vi "FX_Config Extract All.vi"(6 "Send Cmd Timout(ms)":u32=300, 8 "Error":errorcluster, 10 "FX Config":T1={"CAN"={"ID"=0, "Bus"=""}, "Output"={"Inverted"=FALSE, "Neutral"=enum."Override to Coast", "Max"={"FWD"=1.0, "REV"=-1.0}, "Min"={"FWD"=0.0, "REV"=0.0}, "OL Ramp Rate (S)"=0.0, "Dead Band"=0.0, "CL Ramp Rate (S)"=0.0}, "CL"={"Gains"={"P"=1.0, "I"=0.01, "D"=0.0, "F"=0.0}, "Error Allowed"={"High"=0.0, "Low"=0.0}, "I Zone"={"High"=10000.0, "Low"=-1000.0}, "Max Out"={"FWD"=1.0, "REV"=-1.0}, "Max I Accu"={"High"=10.0, "Low"=-10.0}, "CL Ramp Rate (S)"=0.0}, "MM"={"Cruise Velocity"=5000, "Acceleration"=5000}, "TravelLimits"={"Hard"={"FWD Switch Normal"=enum."Normally Open", "FWD On will Zero Encoder "=FALSE, "REV Switch Normal"=enum."Normally Open", "REV On will Zero Encoder "=FALSE}, "Soft"={"FWD"={"Enable"=FALSE, "Counts"=0}, "REV"={"Enable"=FALSE, "Counts"=0}}}, "CurrentLimit"={"Enable"=FALSE, "Current Limit"=0.0, "Threshold Current"=0.0, "Threshold Time"=0.0}} {"TravelLimits"."Soft"."REV"."Counts" format="%#.0f"; "TravelLimits"."Soft"."FWD"."Counts" format="%#.0f"; "Output"."Min"."REV" format="%.2f"; "Output"."Min"."FWD" format="%.2f"; "Output"."Max"."REV" format="%.2f"; "Output"."Max"."FWD" format="%.2f"; "CL"."Max I Accu"."Low" format="%#.8f"; "CL"."Max I Accu"."High" format="%#.8f"; "CL"."Gains"."F" format="%#.8f"; "CL"."Gains"."D" format="%#.8f"; "CL"."Gains"."I" format="%#.8f"; "CL"."Gains"."P" format="%#.8f"; "CL"."Error Allowed"."Low" format="%#.8f"; "CL"."Error Allowed"."High" format="%#.8f"; "CL"."I Zone"."Low" format="%#.8f"; "CL"."I Zone"."High" format="%#.8f"; "CL"."Max Out"."REV" format="%.2f"; "CL"."Max Out"."FWD" format="%.2f"}, 11 "PhoenixMotorControlDevRef":T16={"DeviceStatus"={"status"=FALSE, "code"=0, "source"=""}, "Type"=enum."PWM", "PWM"={"PWM Channel"=enum."Invalid", "DeadBand"={"Name"="", "maxPositivePwm"=0, "minPositivePwm"=0, "centerPwm"=0, "maxNegativePwm"=0, "minNegativePwm"=0, "angularRange"=0}}, "CAN"={"Device Number"=0, "SetOutput VI Ref"=variant, "GetOutput VI Ref"=variant, "Enable VI Ref"=variant, "Disable VI Ref"=variant, "Data"=variant}, "Invert"=FALSE, "DIO PWM"={"PWM \"Enable\" Channel"=enum."Invalid", "DIOChannel"=enum."Invalid", "PWM Rate"=0.0}}) -> (0 "Error Out":errorcluster, 2 "Wrist Config Data Out":T1={"CAN"={"ID"=0, "Bus"=""}, "Output"={"Inverted"=FALSE, "Neutral"=enum."Override to Coast", "Max"={"FWD"=1.0, "REV"=-1.0}, "Min"={"FWD"=0.0, "REV"=0.0}, "OL Ramp Rate (S)"=0.0, "Dead Band"=0.0, "CL Ramp Rate (S)"=0.0}, "CL"={"Gains"={"P"=1.0, "I"=0.01, "D"=0.0, "F"=0.0}, "Error Allowed"={"High"=0.0, "Low"=0.0}, "I Zone"={"High"=10000.0, "Low"=-1000.0}, "Max Out"={"FWD"=1.0, "REV"=-1.0}, "Max I Accu"={"High"=10.0, "Low"=-10.0}, "CL Ramp Rate (S)"=0.0}, "MM"={"Cruise Velocity"=5000, "Acceleration"=5000}, "TravelLimits"={"Hard"={"FWD Switch Normal"=enum."Normally Open", "FWD On will Zero Encoder "=FALSE, "REV Switch Normal"=enum."Normally Open", "REV On will Zero Encoder "=FALSE}, "Soft"={"FWD"={"Enable"=FALSE, "Counts"=0}, "REV"={"Enable"=FALSE, "Counts"=0}}}, "CurrentLimit"={"Enable"=FALSE, "Current Limit"=0.0, "Threshold Current"=0.0, "Threshold Time"=0.0}} {"TravelLimits"."Soft"."REV"."Counts" format="%#.0f"; "TravelLimits"."Soft"."FWD"."Counts" format="%#.0f"; "Output"."Min"."REV" format="%.2f"; "Output"."Min"."FWD" format="%.2f"; "Output"."Max"."REV" format="%.2f"; "Output"."Max"."FWD" format="%.2f"; "CL"."Max I Accu"."Low" format="%#.8f"; "CL"."Max I Accu"."High" format="%#.8f"; "CL"."Gains"."F" format="%#.8f"; "CL"."Gains"."D" format="%#.8f"; "CL"."Gains"."I" format="%#.8f"; "CL"."Gains"."P" format="%#.8f"; "CL"."Error Allowed"."Low" format="%#.8f"; "CL"."Error Allowed"."High" format="%#.8f"; "CL"."I Zone"."Low" format="%#.8f"; "CL"."I Zone"."High" format="%#.8f"; "CL"."Max Out"."REV" format="%.2f"; "CL"."Max Out"."FWD" format="%.2f"}, 3 "Module Azimuth Ref Out":T16)   [LabVIEW 2020]
uses:
  <vilib>/Utility/Data Type/NI_Data Type.lvlib
  <vilib>/Rock Robotics/WPI/ThirdParty/Phoenix-LabVIEW/Motor Controller/Controls/CTRE_Phoenix_MotorControl_LimitSwitchNormal.ctl
  <vilib>/Rock Robotics/WPI/ThirdParty/Phoenix-LabVIEW/Motor Controller/Controls/CTRE_Phoenix_MotorControl_TalonFXInvertType.ctl
  <vilib>/Rock Robotics/WPI/ThirdParty/Phoenix-LabVIEW/Motor Controller/Controls/CTRE_Phoenix_MotorControl_NeutralMode.ctl
  Shared Code/TypeDefs/Cluser_CAN Data.ctl
  Shared Code/TypeDefs/Cluster_FWD  REV Values.ctl
  Shared Code/TypeDefs/Cluster_Config SRX Motor Output.ctl
  Shared Code/TypeDefs/Cluster_PID Gains.ctl
  Shared Code/TypeDefs/Cluster_SRX SLOT PID Config.ctl
  Shared Code/TypeDefs/Cluster_SRX Motion Magic Parameters.ctl
  Shared Code/TypeDefs/Cluser_Hard Limits.ctl
  Shared Code/TypeDefs/Cluser_Enable-Value I32.ctl
  Shared Code/TypeDefs/Cluser_Config_Soft Limits.ctl
  Shared Code/TypeDefs/Cluser_Limit Travel Config.ctl
  Shared Code/TypeDefs/Cluster_Cancoder_Config Data.ctl
  <vilib>/Rock Robotics/SystemInterfaces/DIO/FPGA_DIOPWMChannel.ctl
  <vilib>/Rock Robotics/WPI/PWM/WPI_PWMDeadband.ctl
  <vilib>/Rock Robotics/WPI/MotorControl/WPI_MotorControlType.ctl
  <vilib>/Rock Robotics/SystemInterfaces/DIO/FPGA_DIOChannel.ctl
  <vilib>/Rock Robotics/WPI/MotorControl/WPI_MotorControlDeviceRef.ctl
  Shared Code/TypeDefs/Cluster_High-Low.ctl
  Shared Code/TypeDefs/Cluser_Config_Current Limits.ctl
  Shared Code/TypeDefs/Cluster_FX Config HW Values.ctl
panel:
  # "Tune Output\nto 1023 Max"
  # "Tune Output\nto 1023 Max"
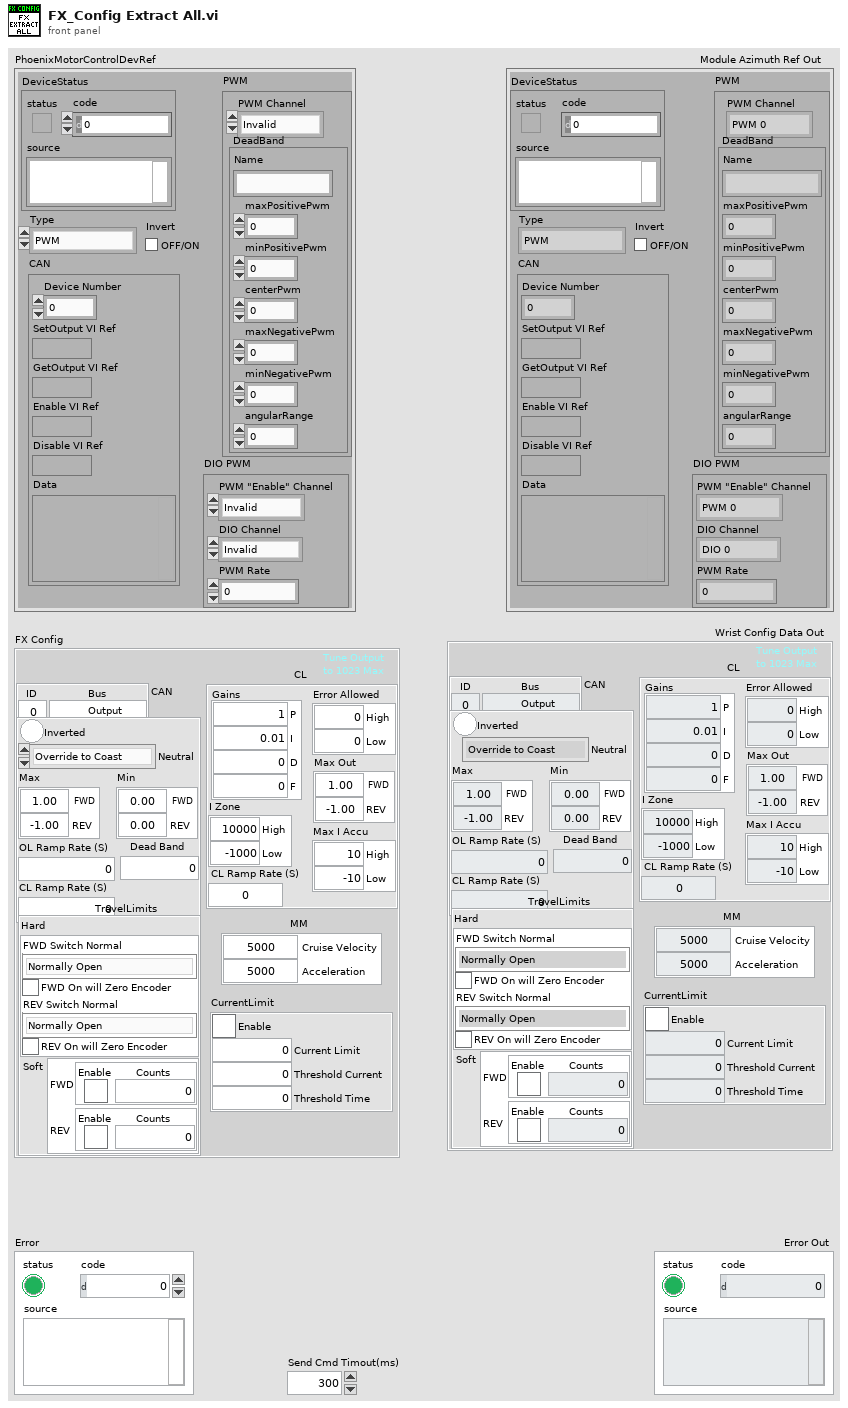
[diagram p1: front panel]
types:
  T1 = typedef "Cluster_FX Config HW Values.ctl" = cluster{"CAN":T2, "Output":T3, "CL":T6, "MM":T9, "TravelLimits":T10, "CurrentLimit":T15}
  T2 = typedef "Cluser_CAN Data.ctl" = cluster{"ID":u8, "Bus":string}
  T3 = typedef "Cluster_Config SRX Motor Output.ctl" = cluster{"Inverted":bool, "Neutral":T4, "Max":T5, "Min":T5, "OL Ramp Rate (S)":dbl, "Dead Band":dbl, "CL Ramp Rate (S)":dbl}
  T4 = typedef "CTRE_Phoenix_MotorControl_NeutralMode.ctl" = enum8{"EEPROMSetting", "Override to Coast", "Override to Brake"}
  T5 = typedef "Cluster_FWD  REV Values.ctl" = cluster{"FWD":dbl, "REV":dbl}
  T6 = typedef "Cluster_PID Config.ctl" = cluster{"Gains":T7, "Error Allowed":T8, "I Zone":T8, "Max Out":T5, "Max I Accu":T8, "CL Ramp Rate (S)":dbl}
  T7 = typedef "Cluster_PID Gains.ctl" = cluster{"P":dbl, "I":dbl, "D":dbl, "F":dbl}
  T8 = typedef "Cluster_High-Low.ctl" = cluster{"High":dbl, "Low":dbl}
  T9 = typedef "Cluster_SRX Motion Magic Parameters.ctl" = cluster{"Cruise Velocity":i32, "Acceleration":i32}
  T10 = typedef "Cluser_Limit Travel Config.ctl" = cluster{"Hard":T11, "Soft":T13}
  T11 = typedef "Cluser_Hard Limits.ctl" = cluster{"FWD Switch Normal":T12, "FWD On will Zero Encoder ":bool, "REV Switch Normal":T12, "REV On will Zero Encoder ":bool}
  T12 = typedef "CTRE_Phoenix_MotorControl_LimitSwitchNormal.ctl" = enum16{"Normally Open", "Normally Closed", "Disabled"}
  T13 = typedef "Cluser_Config_Soft Limits.ctl" = cluster{"FWD":T14, "REV":T14}
  T14 = typedef "Cluser_Enable-Value I32.ctl" = cluster{"Enable":bool, "Counts":i32}
  T15 = typedef "Cluser_Config_Current Limits.ctl" = cluster{"Enable":bool, "Current Limit":dbl, "Threshold Current":dbl, "Threshold Time":dbl}
  T16 = typedef "WPI_MotorControlDeviceRef.ctl" = cluster{"DeviceStatus":errorcluster, "Type":T17, "PWM":cluster{"PWM Channel":T18, "DeadBand":T19}, "CAN":cluster{"Device Number":u8, "SetOutput VI Ref":variant, "GetOutput VI Ref":variant, "Enable VI Ref":variant, "Disable VI Ref":variant, "Data":variant}, "Invert":bool, "DIO PWM":cluster{"PWM \"Enable\" Channel":T18, "DIOChannel":T20, "PWM Rate":dbl}}
  T17 = typedef "WPI_MotorControlType.ctl" = enum16{"PWM", "CAN", "DIO PWM"}
  T18 = typedef "FPGA_DIOPWMChannel.ctl" = enum8{"PWM 0", "PWM 1", "PWM 2", "PWM 3", "PWM 4", "PWM 5", "PWM 6", "PWM 7", "PWM 8", "PWM 9", "PWM MXP 0", "PWM MXP 1", "PWM MXP 2", "PWM MXP 3", "PWM MXP 4", "PWM MXP 5", "PWM MXP 6", "PWM MXP 7", "PWM MXP 8", "PWM MXP 9", "Invalid"}
  T19 = typedef "WPI_PWMDeadband.ctl" = cluster{"Name":string, "maxPositivePwm":i32, "minPositivePwm":i32, "centerPwm":i32, "maxNegativePwm":i32, "minNegativePwm":i32, "angularRange":u16}
  T20 = typedef "FPGA_DIOChannel.ctl" = enum8{"DIO 0", "DIO 1", "DIO 2", "DIO 3", "DIO 4", "DIO 5", "DIO 6", "DIO 7", "DIO 8", "DIO 9", "DIO MXP 0", "DIO MXP 1", "DIO MXP 2", "DIO MXP 3", "DIO MXP 4", "DIO MXP 5", "DIO MXP 6", "DIO MXP 7", "DIO MXP 8", "DIO MXP 9", "DIO MXP 10", "DIO MXP 11", "DIO MXP 12", "DIO MXP 13", "DIO MXP 14", "DIO MXP 15", "SPI Port CS1", "SPI Port CS2", "SPI Port CS3", "SPI Port MISO", "SPI Port MOSI", "Invalid"}
  T21 = typedef "Cluster_Cancoder_Config Data.ctl" = cluster{"ID":u8, "CW(t) CCW(f)":bool, "Zero Offset":dbl}
  T22 = typedef "Cluster_SRX SLOT PID Config.ctl" = cluster{"Gains":T7, "Error Allowed":dbl, "I Zone":dbl, "Peak Out 0-1":dbl, "Max I Accu":dbl}
  T23 = typedef "Cluster_Config SRX Motor Output.ctl" = cluster{"Neutral":T4, "Max":T5, "Min":T5, "OL Ramp Rate (S)":dbl, "Dead Band":dbl, "CL Ramp Rate (S)":dbl}
  T24 = typedef "CTRE_Phoenix_MotorControl_TalonFXInvertType.ctl" = enum16{"Counter-Clockwise", "Clockwise"}
  T25 = typedef "CTRE_Phoenix_MotorControl_TalonFXMotorControllerConfigurables.ctl" = cluster{"Base Configurables":T26, "primaryPID":cluster{"selectedFeedbackCoefficient":dbl, "selectedFeedbackSensor":T32}, "auxiliaryPID":cluster{"selectedFeedbackCoefficient":dbl, "selectedFeedbackSensor":T32}, "forwardLimitSwitchNormal":T12, "reverseLimitSwitchNormal":T12, "forwardLimitSwitchDeviceID":i32, "reverseLimitSwitchDeviceID":i32, "forwardLimitSwitchSource":T33, "reverseLimitSwitchSource":T33, "sum0Term":T32, "sum1Term":T32, "diff0Term":T32, "diff1Term":T32, "Supply Current Limit Configuration":T34, "Stator Current Limit Configuration":T35, "Motor Commutation":T36, "Absolute Sensor Range":T37, "Integrated Sensor Offset (Degrees)":dbl, "Sensor Initialization Strategy":T38}
  T26 = typedef "CTRE_Phoenix_MotorControl_BaseConfigurables.ctl" = cluster{"openLoopRamp":dbl, "closedLoopRamp":dbl, "peakOutputForward":dbl, "peakOutputReverse":dbl, "nominalOutputForward":dbl, "nominalOutputReverse":dbl, "neutralDeadband":dbl, "voltageCompSaturation":dbl, "voltageMeasurementFilter":i32, "velocityMeasurementPeriod":T27, "velocityMeasurementWindow":i32, "forwardSoftLimitThreshold":i32, "reverseSoftLimitThreshold":i32, "forwardSoftLimitEnable":bool, "reverseSoftLimitEnable":bool, "slot0":T28, "slot1":T28, "slot2":T28, "slot3":T28, "auxPIDPolarity":bool, "remoteFilter0":T29, "remoteFilter1":T29, "motionCruiseVelocity":i32, "motionAcceleration":i32, "motionProfileTrajectoryPeriod":i32, "feedbackNotContinuous":bool, "remoteSensorClosedLoopDisableNeutralOnLOS":bool, "clearPositionOnLimitF":bool, "clearPositionOnLimitR":bool, "clearPositionOnQuadIdx":bool, "limitSwitchDisableNeutralOnLOS":bool, "softLimitDisableNeutralOnLOS":bool, "pulseWidthPeriod_EdgesPerRot":i32, "pulseWidthPeriod_FilterWindowSz":i32, "customParam":T31, "trajectoryInterpolationEnable":bool}
  T27 = typedef "CTRE_Phoenix_MotorControl_VelocityMeasurementPeriod.ctl" = u16
  T28 = typedef "CTRE_Phoenix_MotorControl_SlotStructure.ctl" = cluster{"P":dbl, "I":dbl, "D":dbl, "F":dbl, "integralZone":dbl, "allowableClosedLoopError":i32, "maxIntegralAccumulator":dbl, "closedLoopPeakOutput":dbl, "closedLoopPeriod":i32}
  T29 = typedef "CTRE_Phoenix_MotorControl_FilterStruct.ctl" = cluster{"remoteSensorDeviceID":u8, "remoteSensorSource":T30}
  T30 = typedef "CTRE_Phoenix_MotorControl_RemoteSourceType.ctl" = enum16{"Off", "Talon SRX Selected Sensor", "Pigeon IMU Yaw", "Pigeon IMU Pitch", "Pigeon IMU Roll", "CANifier Quadrature", "CANifier PWM Input 0", "CANifier PWM Input 1", "CANifier PWM Input 2", "CANifier PWM Input 3", "Gadgeteer Pigeon Yaw", "Gadgeteer Pigeon Pitch", "Gadgeteer Pigeon Roll", "CANCoder"}
  T31 = typedef "CTRE_Phoenix_CustomParamConfiguration.ctl" = cluster{"customParam0":i32, "customParam1":i32}
  T32 = typedef "CTRE_Phoenix_MotorControl_FeedbackDevice_TalonFX.ctl" = i8
  T33 = typedef "CTRE_Phoenix_MotorControl_LimitSwitchSource_Local.ctl" = enum16{"Feedback Connector", "Remote Talon SRX", "Remote CANifier", "Deactivated"}
  T34 = typedef "CTRE_Phoenix_MotorControl_SupplyCurrentLimitConfiguration.ctl" = cluster{"Enable?":bool, "Current Limit":dbl, "Threshold Current":dbl, "Threshold Time":dbl}
  T35 = typedef "CTRE_Phoenix_MotorControl_StatorCurrentLimitConfiguration.ctl" = cluster{"Enable?":bool, "Current Limit":dbl, "Threshold Current":dbl, "Threshold Time":dbl}
  T36 = typedef "CTRE_Phoenix_MotorControl_MotorCommutation_TalonFX.ctl" = enum16{"Trapezoidal"}
  T37 = typedef "CTRE_Phoenix_CANcoder_AbsoluteSensorRange.ctl" = enum16{"Unsigned [0 to 360)", "Signed [-180 to +180)"}
  T38 = typedef "CTRE_Phoenix_CANcoder_SensorInitializationStrategy.ctl" = enum16{"Boot To Zero", "Boot To Absolute Position"}
  T39 = typedef "Cluster_Config FX Motor Output.ctl" = cluster{"Type":T24, "Neutral":T4, "Max":T5, "Min":T5, "OL Ramp Rate (S)":dbl, "Dead Band":dbl, "CL Ramp Rate (S)":dbl}
  T40 = typedef "Cluster_FX SLOT PID Config.ctl" = cluster{"Gains":T7, "Error Allowed":dbl, "I Zone":dbl, "Peak Out 0-1":dbl, "Max I Accu":dbl}
  T41 = typedef "Cluster_Motion Magic Parameters.ctl" = cluster{"Cruise Velocity":i32, "Acceleration":i32}
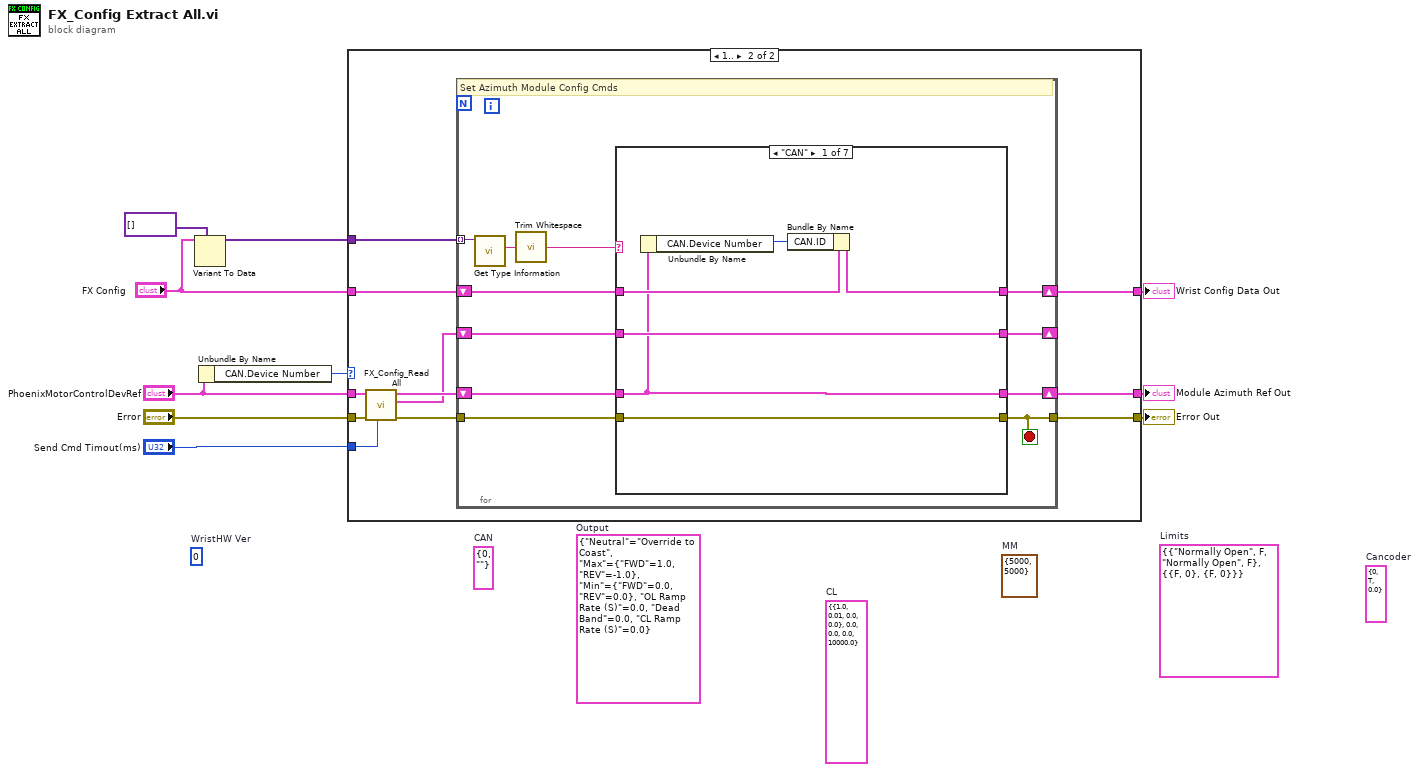
[diagram p0: block diagram]
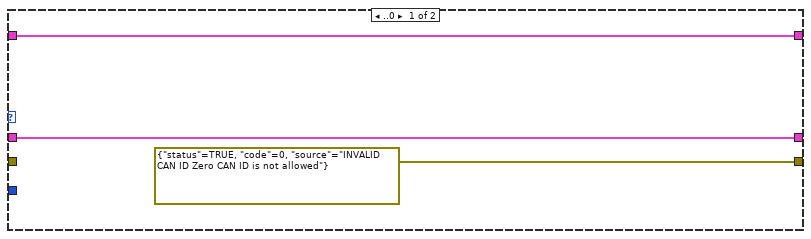
[diagram p2: hidden frame]
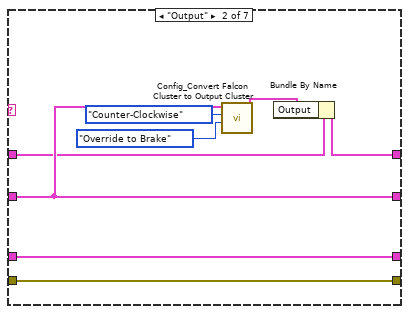
[diagram p3: hidden frame]
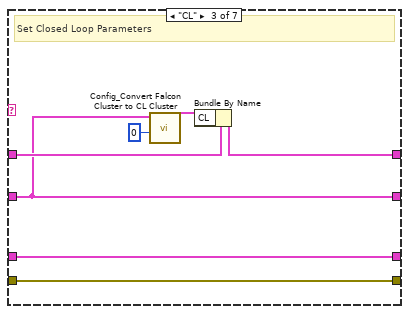
[diagram p4: hidden frame]
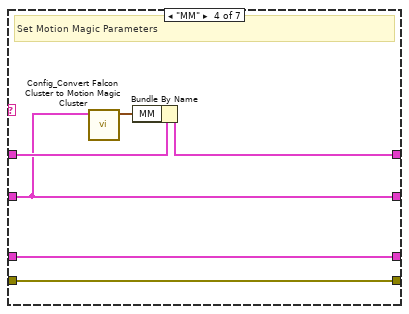
[diagram p5: hidden frame]
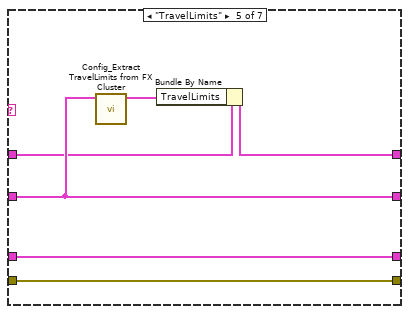
[diagram p6: hidden frame]
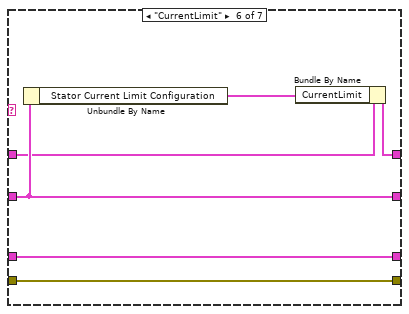
[diagram p7: hidden frame]
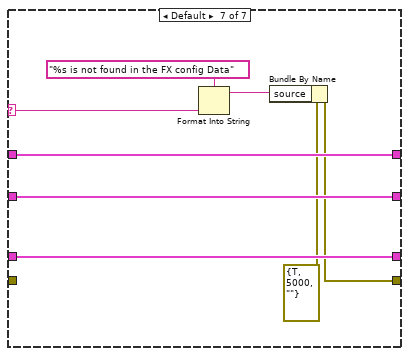
[diagram p8: hidden frame]
diagram:
  (unwired) T21 {"ID"=0, "CW(t) CCW(f)"=TRUE, "Zero Offset"=0.0}  # Cancoder
  (unwired) T10 {"Hard"={"FWD Switch Normal"=enum."Normally Open", "FWD On will Zero Encoder "=FALSE, "REV Switch Normal"=enum."Normally Open", "REV On will Zero Encoder "=FALSE}, "Soft"={"FWD"={"Enable"=FALSE, "Counts"=0}, "REV"={"Enable"=FALSE, "Counts"=0}}}  # Limits
  (unwired) T9 {"Cruise Velocity"=5000, "Acceleration"=5000}  # MM
  (unwired) T22 {"Gains"={"P"=1.0, "I"=0.01, "D"=0.0, "F"=0.0}, "Error Allowed"=0.0, "I Zone"=0.0, "Peak Out 0-1"=0.0, "Max I Accu"=10000.0}  # CL
  (unwired) T23 {"Neutral"=enum."Override to Coast", "Max"={"FWD"=1.0, "REV"=-1.0}, "Min"={"FWD"=0.0, "REV"=0.0}, "OL Ramp Rate (S)"=0.0, "Dead Band"=0.0, "CL Ramp Rate (S)"=0.0}  # Output
  (unwired) T2 {"ID"=0, "Bus"=""}  # CAN
  (unwired) u64 0  # WristHW Ver
  n1 = Variant To Data(type=variant[] [], Variant="FX Config") -> (data=w5:variant[])  [unwired: 1 in, 1 out]
  n2 = Unbundle By Name("PhoenixMotorControlDevRef") -> ("CAN.Device Number"=w1:u8)
  n3 = case shown="1.." w1 {
    tunnel: [w13 w24] -> w10
    tunnel: [errorcluster {"status"=TRUE, "code"=0, "source"="INVALID CAN ID Zero CAN ID is not allowed"} ("Error Out") w23] -> w9
    tunnel: "FX Config" -> [w11 w22]
    tunnel: [w11 w21] -> w6
    tunnel: w5 -> [_ w20]
    tunnel: "Error" -> [_ w19]
    tunnel: "Send Cmd Timout(ms)" -> [_ w16]
    tunnel: "PhoenixMotorControlDevRef" -> [w13 w15]
    frame ..0 {
    }
    frame 1.. {
      n4 = call "FX_Config_Read All.vi"("Send Cmd Timout(ms)"=w16, "Error"=w19, "PhoenixMotorControlDevRef"=w15) -> ("Error Out"=w18:errorcluster, "FX Config Out"=w14:T25, "Ref Out"=w17:T16)  [unwired: 6 in]
      n5 = for {
        shift-right: [w35] -> w24
        shift-left: w17 -> [w33]
        tunnel: w20 -> [w32] mode=indexing
        tunnel: w18 -> [w25]
        tunnel: [w30] -> w23
        shift-right: [w31] -> w21
        shift-left: w22 -> [w34]
        shift-right: [w29] -> _
        shift-left: w14 -> [w28]
        stop <- w30 stop-if-true
        # "Set Azimuth Module Config Cmds"
        n6 = call <vilib>:"Get Type Information.vi"("variant"=w32) -> ("name"=w27:string)  [unwired: 6 in, 4 out]
        n7 = call <vilib>:"Trim Whitespace.vi"("string"=w27) -> ("trimmed string"=w26:string)  [unwired: 1 in]
        n8 = case shown="\"CAN\"" w26 {
          selector: w26 -> [_ _ _ _ _ _ w79]
          tunnel: [w41 w49 w55 w59 w68 w69 w76] -> w30
          tunnel: w33 -> [w37 w48 w56 w60 w67 w74 w82]
          tunnel: [w37 w48 w56 w60 w67 w74 w82] -> w35
          tunnel: w34 -> [w38 w42 w54 w61 w64 w72 w81]
          tunnel: [w39 w43 w53 w62 w65 w71 w81] -> w31
          tunnel: [w40 w47 w50 w58 w66 w73 w80] -> w29
          tunnel: w28 -> [w40 w47 w50 w58 w66 w73 w80]
          tunnel: w25 -> [w41 w49 w55 w59 w68 w69 _]
          frame "CAN" {
            n9 = Unbundle By Name(w37) -> ("CAN.Device Number"=w36:u8)
            n10 = Bundle By Name(cluster=w38, "CAN.ID"=w36) -> (w39:T1)
          }
          frame "Output" {
            n11 = call "Config_Convert Falcon Cluster to Output Cluster.vi"("Neutral Mode"=CTRE_Phoenix_MotorControl_NeutralMode."Override to Brake", "Rotation Type"=CTRE_Phoenix_MotorControl_TalonFXInvertType."Counter-Clockwise", "Talon FX Configurables"=w47) -> ("Motor Output Out"=w44:T39)  [unwired: 8 in]
            n12 = Bundle By Name(cluster=w42, "Output"=w44) -> (w43:T1)
          }
          frame "CL" {
            # "Set Closed Loop Parameters"
            n13 = call "Config_Convert Falcon Cluster to CL Cluster.vi"("Slot"=0, "Talon FX Configurables"=w50) -> ("CL"=w52:T40)  [unwired: 8 in, 1 out]
            n14 = Bundle By Name(cluster=w54, "CL"=w52) -> (w53:T1)
          }
          frame "MM" {
            # "Set Motion Magic Parameters"
            n15 = call "Config_Convert Falcon Cluster to Motion Magic Cluster.vi"("Talon FX Configurables"=w58) -> ("MM"=w57:T41)  [unwired: 10 in]
            n16 = Bundle By Name(cluster=w61, "MM"=w57) -> (w62:T1)
          }
          frame "TravelLimits" {
            n17 = call "Config_Extract TravelLimits from FX Cluster.vi"("Talon FX Configurables"=w66) -> ("Limits Out"=w63:T10)  [unwired: 10 in]
            n18 = Bundle By Name(cluster=w64, "TravelLimits"=w63) -> (w65:T1)
          }
          frame "CurrentLimit" {
            n19 = Unbundle By Name(w73) -> ("Stator Current Limit Configuration"=w70:T35)
            n20 = Bundle By Name(cluster=w72, "CurrentLimit"=w70) -> (w71:T1)
          }
          frame Default {
            n21 = Format Into String(format string="%s is not found in the FX config Data", w79) -> (resulting string=w75:string)  [unwired: 2 in, 1 out]
            n22 = Bundle By Name(cluster=errorcluster {"status"=TRUE, "code"=5000, "source"=""} ("Error Out"), "source"=w75) -> (w76:errorcluster)
          }
        }
      }
    }
  }
  "Module Azimuth Ref Out" <- w10
  "Error Out" <- w9
  "Wrist Config Data Out" <- w6
